vi "Get Filter Wheel Positions.vi"(8 "error in (no error)":errorcluster) -> (0 "error out":errorcluster, 3 "Filter Wheels":string[](array[string]))   [LabVIEW 2021]
uses:
  Logging/CC enum Current Values Action.ctl
  hk-channel-class/HK Table/HK Table.lvclass
  Filter Wheel/Filter Wheel Object/Filter Wheel.lvclass
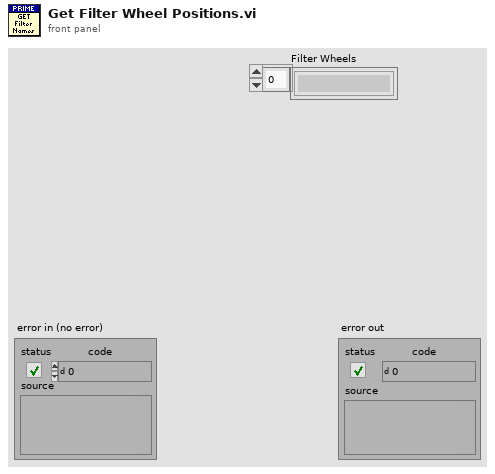
[diagram p1: front panel]
types:
  T1 = typedef "CC enum Current Values Action.ctl" = enum16{"Init", "Write Item", "Write Array", "Read Item", "Read Array", "Read All", "Add Channels", "New File", "Add Message", "Get Current Values", "Close"}
  T2 = typedef "Filter Wheel.lvclass/Filter Wheel configuration.ctl" = cluster{"Num Wheels":i32, "Filters":T3[], "Invalid Combinations":i32[][], "Addr":refnum<visa-resource-name>, "Name":string, "Simulate":bool, "Homing Parameters":T4, "Default Speed":u16}
  T3 = typedef "Filter Wheel.lvclass/Filter Wheel Details.ctl" = cluster{"Names":string[], "Relative Position":i32[], "Wheel Name":string}
  T4 = typedef "Filter Wheel Arduino Homing cluster.ctl" = cluster{"Direction (F: CW)":bool, "Speed":i32, "Accel":i32, "Min Distance":i32, "Short Leg":i32, "Error Cnts":i32}
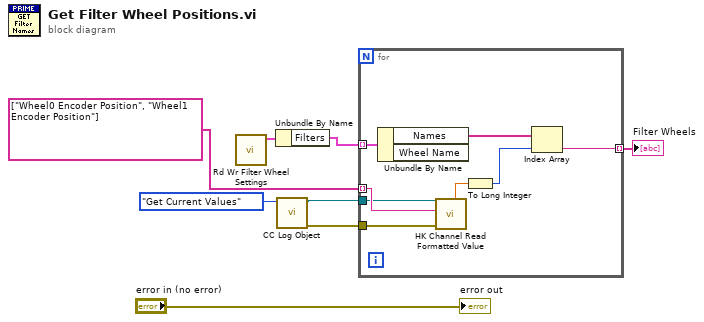
[diagram p0: block diagram]
diagram:
  n1 = call "Rd Wr Filter Wheel Settings.vi"() -> ("Filter Wheel Settings"=w6:T2)  [unwired: 10 in, 1 out]
  n2 = Unbundle By Name(w6) -> ("Filters"=w2:T3[])
  n3 = call "CC Log Object.vi"("Action"=CC_enum_Current_Values_Action."Get Current Values") -> ("error out"=w4:errorcluster, "HK Channel out"=w3:refnum<class "HK Table.lvclass">)  [unwired: 8 in, 1 out]
  n4 = for {
    tunnel: string[] ["Wheel0 Encoder Position", "Wheel1 Encoder Position"] -> [w13] mode=indexing
    tunnel: w4 -> [w12]
    tunnel: w3 -> [w11]
    tunnel: w2 -> [w10] mode=indexing
    tunnel: [w9] -> w1 mode=indexing
    n5 = Unbundle By Name(w10) -> ("Names"=w15:string[])  [unwired: 1 out]
    n6 = call-dynamic "HK Channel Read Formatted Value.vi"("error in (no error)"=w12, "Name"=w13, "HK Channel in"=w11) -> ("Value"=w16:dbl)  [unwired: 1 in, 7 out]
    n7 = To Long Integer(number=w16) -> (32bit integer=w14:i32)
    n8 = Index Array(array=w15, index=w14) -> (element=w9:string)
  }
  "Filter Wheels" <- w1
  "error out" <- "error in (no error)"
